vi "Global 1.vi"() -> ()   [LabVIEW 2020]
panel:
  in  "Stop Media":bool
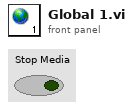
[diagram p1: front panel]
diagram:
